vi "RD_array_result.vi"(7 "Offset array":dbl[](array[numeric]), 8 "lower limit":dbl=2.1 format="%#_13g", 9 "upper limit":dbl, 11 "Input":dbl[](array[numeric])) -> (0 "data":T1, 1 "結果":bool, 2 "字串":string, 3 "數據結果":string, 4 "數據":dbl[](array[numeric]))   [LabVIEW 2019]
panel:
  out "超過範圍NG":bool[](array[boolean])
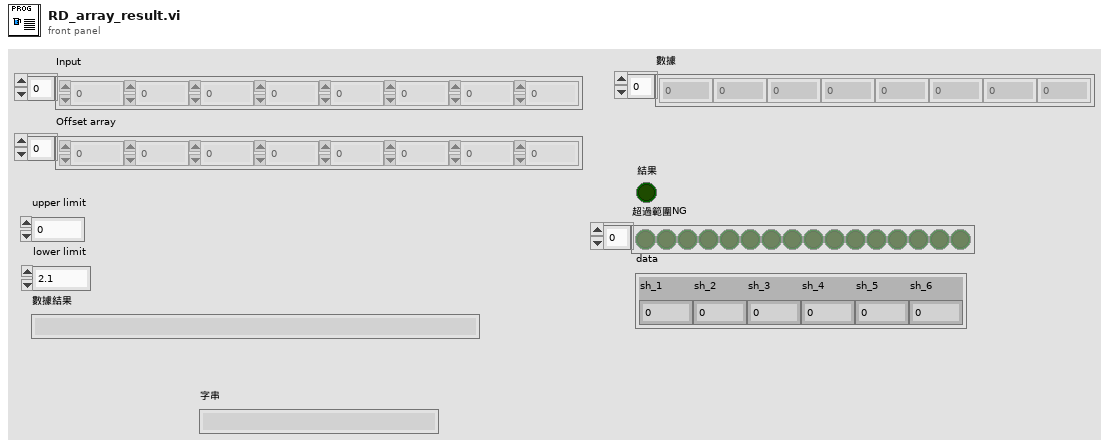
[diagram p1: front panel]
types:
  T1 = cluster{"sh_1":dbl, "sh_2":dbl, "sh_3":dbl, "sh_4":dbl, "sh_5":dbl, "sh_6":dbl}
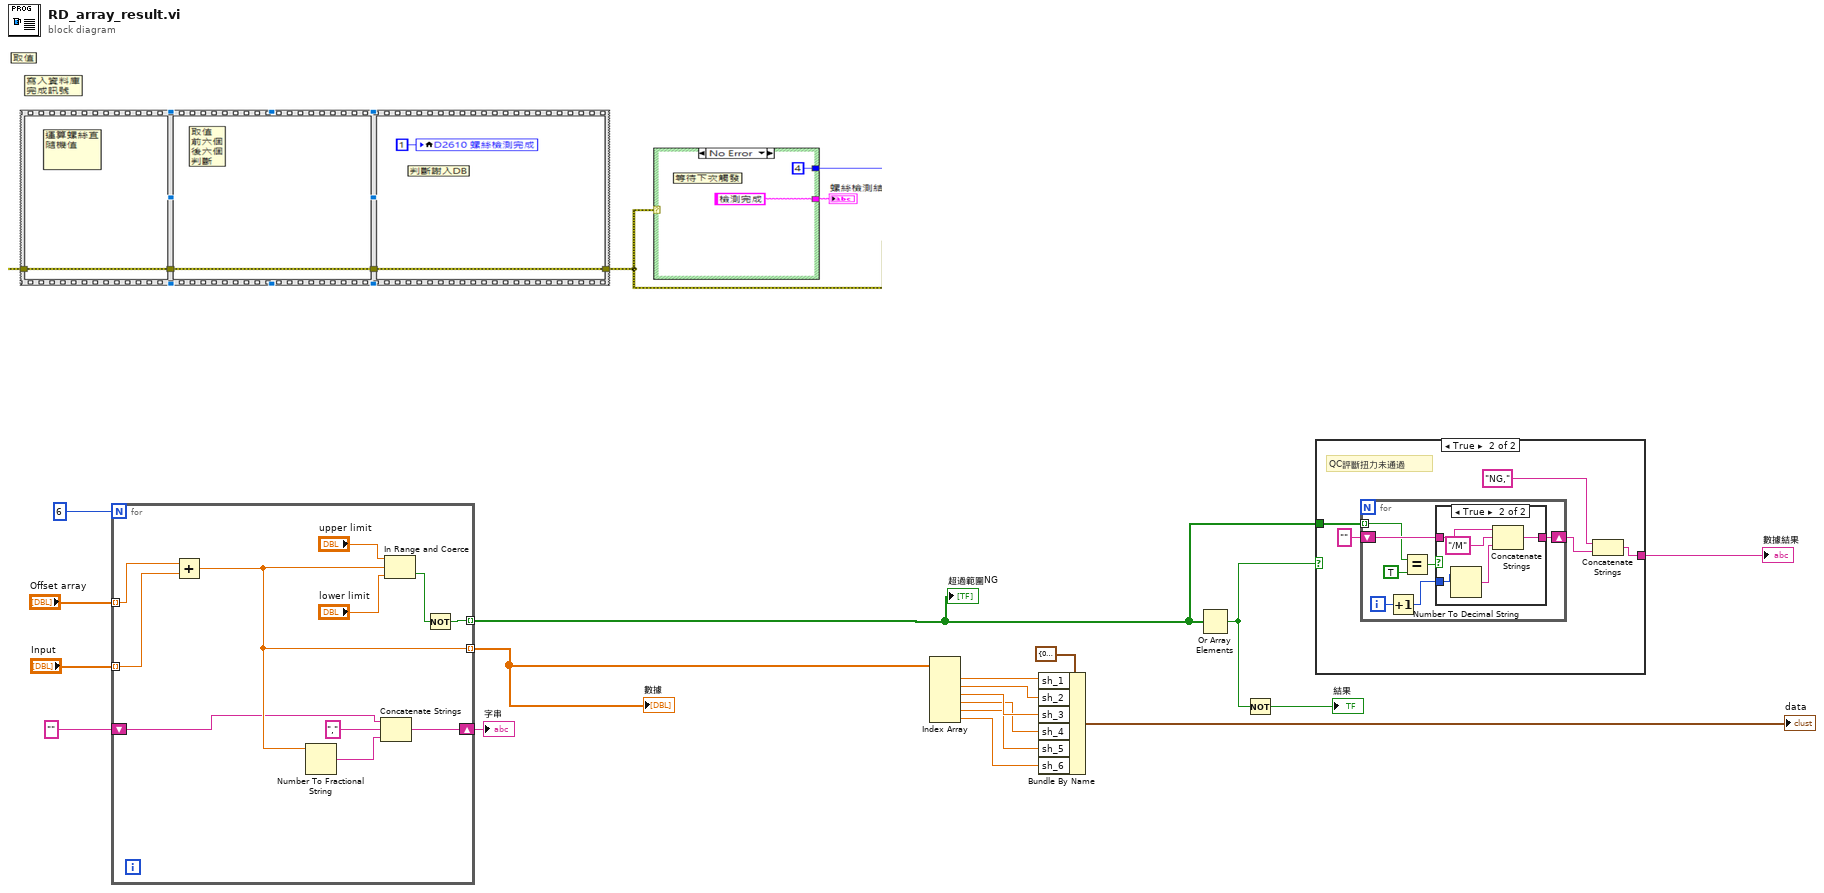
[diagram p0: block diagram]
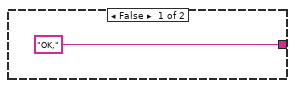
[diagram p2: hidden frame]
diagram:
  n1 = for {
    N: 6 -> [_]
    tunnel: [w26] -> w5 mode=indexing
    tunnel: [w25] -> w17 mode=indexing
    shift-right: [w21] -> w3
    shift-left: "" -> [w22]
    tunnel: "Offset array" -> [w20] mode=indexing
    tunnel: "Input" -> [w19] mode=indexing
    n2 = Add(x=w20, y=w19) -> (x+y=w25:dbl)
    n3 = Number To Fractional String(number=w25) -> (F-format string=w23:string)  [unwired: 3 in]
    n4 = Concatenate Strings(w22, "," ("string"), w23) -> (w21:string)
    n5 = In Range and Coerce(upper limit="upper limit", x=w25, lower limit="lower limit") -> (In Range?=w27:bool)  [unwired: 1 out]
    n6 = Not(x=w27) -> (.not. x?=w26:bool)
  }
  "超過範圍NG" <- w5
  "字串" <- w3
  "數據" <- w17
  n7 = Index Array(array=w17) -> (element #1=w15:dbl, element #2=w14:dbl, element #3=w13:dbl, element #4=w12:dbl, element #5=w11:dbl, element #6=w10:dbl)  [unwired: 6 in]
  n8 = Bundle By Name(cluster=T1 {"sh_1"=0.0, "sh_2"=0.0, "sh_3"=0.0, "sh_4"=0.0, "sh_5"=0.0, "sh_6"=0.0}, "sh_1"=w15, "sh_2"=w14, "sh_3"=w13, "sh_4"=w12, "sh_5"=w11, "sh_6"=w10) -> (→"data":T1)
  n9 = Or Array Elements(Boolean array=w5) -> (logical OR=w2:bool)
  n10 = Not(x=w2) -> (.not. x?=→"結果":bool)
  n11 = case shown="True" w2 {
    tunnel: ["OK," ("screw_result") w33] -> w4
    tunnel: w5 -> [_ w35]
    frame False {
    }
    frame True {
      # "QC評斷扭力未通過"
      n12 = for {
        tunnel: w35 -> [w40] mode=indexing
        shift-right: [w36] -> w34
        shift-left: "" -> [w42]
        i -> [w38]
        n13 = Increment(x=w38) -> (x+1=w37:i32)
        n14 = Equal?(x=w40, y=TRUE) -> (x = y?=w39:bool)
        n15 = case shown="True" w39 {
          tunnel: w42 -> [w43 w48]
          tunnel: w37 -> [_ w46]
          tunnel: [w43 w44] -> w36
          frame False {
          }
          frame True {
            n16 = Number To Decimal String(number=w46) -> (decimal integer string=w45:string)  [unwired: 1 in]
            n17 = Concatenate Strings(w48, "/M" ("string"), w45) -> (w44:string)
          }
        }
      }
      n18 = Concatenate Strings("NG,", w34) -> (w33:string)
    }
  }
  "數據結果" <- w4
